vi "_findOpenStorage.vi"(4 "error in (no error)":errorcluster, 6 "Storage type":string="USI", 7 "Storage location":path) -> (0 "error out":errorcluster, 3 "storage refnum":refnum<k20>)   [LabVIEW 2020]
uses:
  <resource>/objmgr/Storage.rc
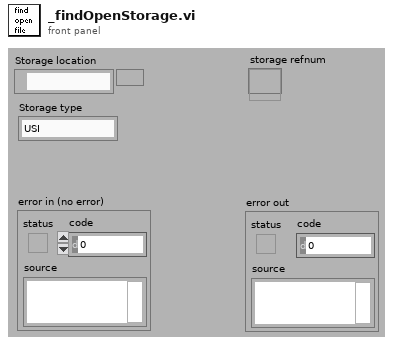
[diagram p1: front panel]
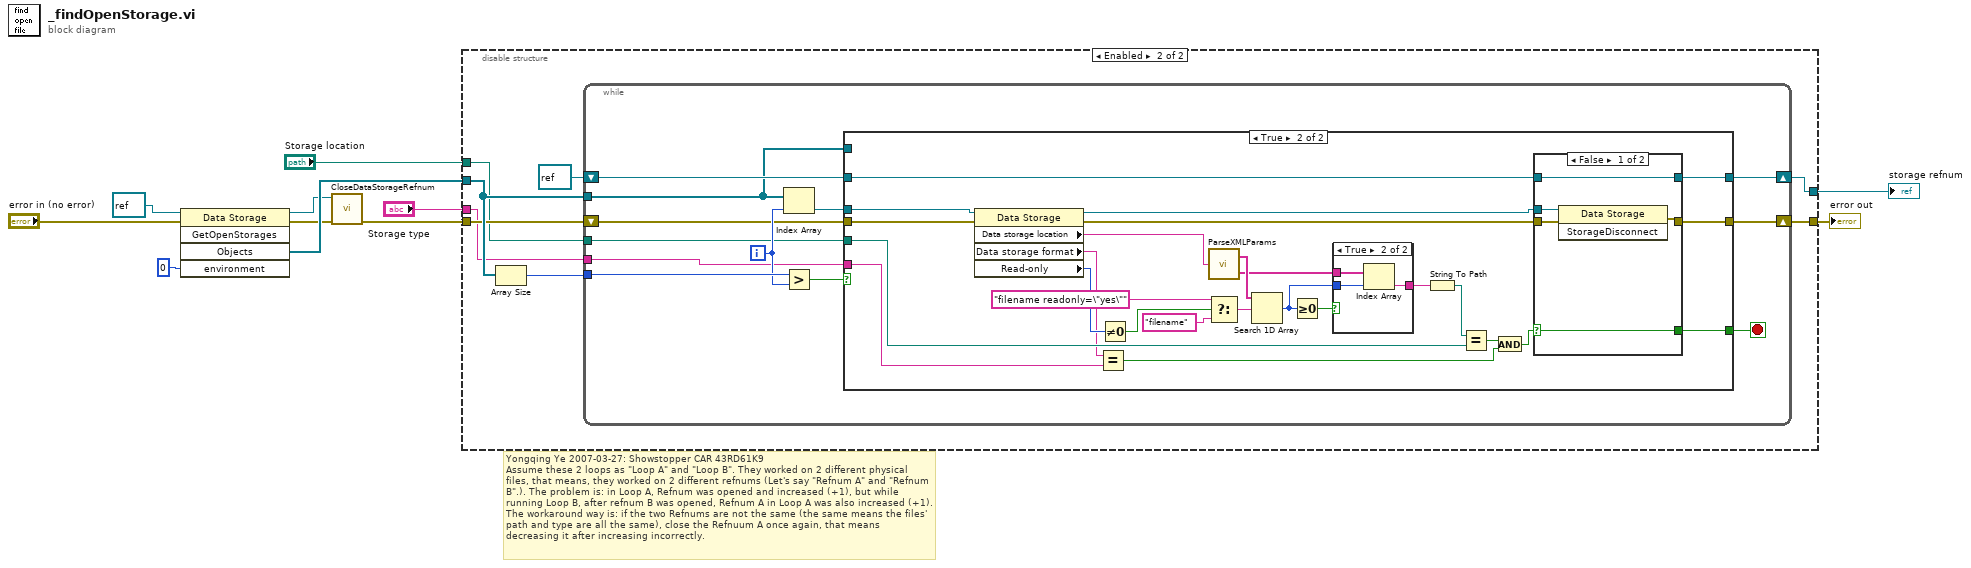
[diagram p0: block diagram]
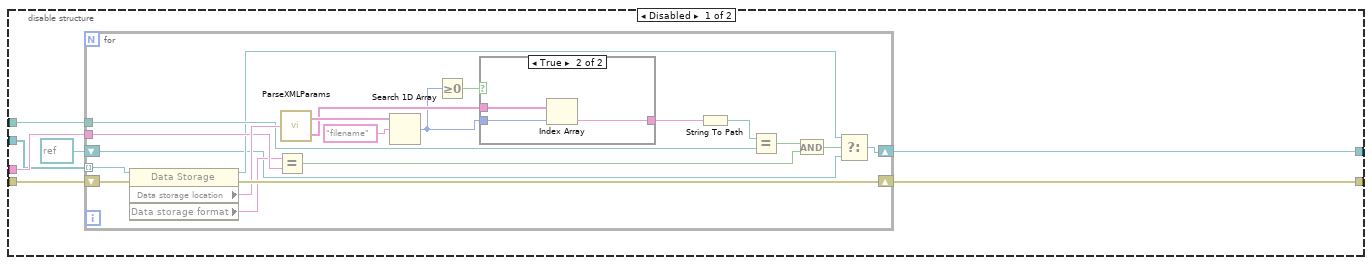
[diagram p2: hidden frame]
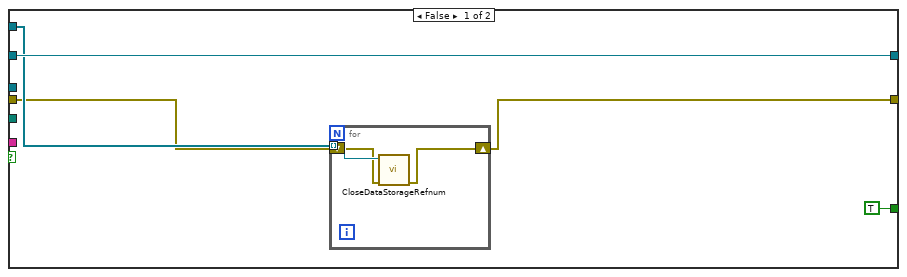
[diagram p4: hidden frame]
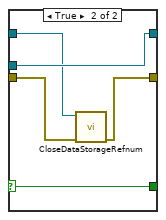
[diagram p6: hidden frame]
diagram:
  # "Yongqing Ye 2007-03-27: Showstopper CAR 43RD61K9\nAssume these 2 loops as \"Loop A\" and \"Loop B\". They worked on 2 different physical files, that means, they worked on 2 different refnums (Let's say \"Refnum A\" and \"Refnum B\".). The problem is: in Loop A, Refnum was opened and increased (+1), but while running Loop B, after refnum B was opened, Refnum A in Loop A was also increased (+1). The workaround way is: if the two Refnums are not the same (the same means the files' path and type are all the same), close the Refnuum A once again, that means decreasing it after increasing incorrectly."
  n1 = invoke class="Data Storage" method="GetOpenStorages"(reference=refnum<k20> refnum, error in="error in (no error)", "environment"=0) -> (reference out=w3:refnum<k20>, error out=w2:errorcluster, "Objects"=w6:refnum<k20>[])  [unwired: 2 in, 2 out]
  n2 = call "CloseDataStorageRefnum.vi"("error in (no error)"=w2, "reference"=w3) -> ("error out"=w1:errorcluster)  [unwired: 9 in]
  n3 = disable-structure shown="Enabled" {
    disable-tunnel: [w18 w42] -> w11
    disable-tunnel: "Storage type" -> [w17 w44]
    disable-tunnel: "Storage location" -> [w16 w45]
    disable-tunnel: [w15 w43] -> w7
    disable-tunnel: w1 -> [w14 w46]
    disable-tunnel: w6 -> [w13 w48]
    frame Disabled {
      n4 = for {
        tunnel: w13 -> [w38] mode=indexing
        shift-right: [w36] -> w18
        shift-left: w14 -> [w37]
        tunnel: w16 -> [w27]
        tunnel: w17 -> [w26]
        shift-right: [w19] -> w15
        shift-left: refnum<k20> refnum ("reference") -> [w20]
        n5 = property class="Data Storage"(reference=w38, error in=w37) -> (reference out=w21:refnum<k20>, error out=w36:errorcluster, "Data storage location"=w30:string, "Data storage format"=w25:string)
        n6 = Equal?(x=w25, y=w26) -> (x = y?=w24:bool)
        n7 = call "ParseXMLParams.vi"("Parameter String"=w30) -> ("Names"=w35:string[], "Values"=w32:string[])
        n8 = Search 1D Array(1D array=w35, element="filename") -> (index of element=w31:i32)  [unwired: 1 in]
        n9 = Greater Or Equal To 0?(x=w31) -> (x >= 0?=w33:bool)
        n10 = case shown="True" w33 {
          tunnel: w32 -> [_ w41]
          tunnel: w31 -> [_ w40]
          tunnel: [_ w39] -> w29
          frame False {
          }
          frame True {
            n11 = Index Array(array=w41, index=w40) -> (element=w39:string)
          }
        }
        n12 = String To Path(string=w29) -> (path=w28:path)
        n13 = Equal?(x=w28, y=w27) -> (x = y?=w23:bool)
        n14 = And(x=w23, y=w24) -> (x .and. y?=w22:bool)
        n15 = Select(t=w21, s=w22, f=w20) -> (s? t:f=w19:refnum<k20>)
      }
    }
    frame Enabled {
      n16 = Array Size(array=w48) -> (size(s)=w49:i32)
      n17 = while {
        tunnel: w49 -> [w61]
        tunnel: w48 -> [w50]
        shift-right: [w51] -> w43
        shift-left: refnum<k20> refnum ("reference") -> [w57]
        tunnel: w45 -> [w55]
        tunnel: w44 -> [w54]
        shift-right: [w52] -> w42
        shift-left: w46 -> [w56]
        i -> [w59]
        stop <- w53 stop-if-true
        n18 = Index Array(array=w50, index=w59) -> (element=w58:refnum<k20>)
        n19 = Greater?(x=w61, y=w59) -> (0:w60:bool)
        n20 = case shown="True" w60 {
          tunnel: w58 -> [_ w76]
          tunnel: w57 -> [w65 w89]
          tunnel: w56 -> [w63 w75]
          tunnel: w55 -> [_ w93]
          tunnel: w54 -> [_ w92]
          tunnel: [TRUE w87] -> w53
          tunnel: [w62 w88] -> w52
          tunnel: [w65 w90] -> w51
          tunnel: w50 -> [w64 _]
          frame False {
            n21 = for {
              tunnel: w64 -> [w69] mode=indexing
              shift-right: [w67] -> w62
              shift-left: w63 -> [w68]
              n22 = call "CloseDataStorageRefnum.vi"("error in (no error)"=w68, "reference"=w69) -> ("error out"=w67:errorcluster)  [unwired: 9 in]
            }
          }
          frame True {
            n23 = property class="Data Storage"(reference=w76, error in=w75) -> (reference out=w74:refnum<k20>, error out=w73:errorcluster, "Data storage location"=w72:string, "Data storage format"=w70:string, "Read-only"=w71:i32)
            n24 = Equal?(x=w70, y=w92) -> (x = y?=w95:bool)
            n25 = Not Equal To 0?(x=w71) -> (x != 0?=w79:bool)
            n26 = call "ParseXMLParams.vi"("Parameter String"=w72) -> ("Names"=w86:string[], "Values"=w84:string[])
            n27 = Select(t="filename readonly=\"yes\"", s=w79, f="filename" ("element")) -> (s? t:f=w80:string)
            n28 = Search 1D Array(1D array=w86, element=w80) -> (index of element=w83:i32)  [unwired: 1 out]
            n29 = Greater Or Equal To 0?(x=w83) -> (x >= 0?=w85:bool)
            n30 = case shown="True" w85 {
              tunnel: w84 -> [_ w98]
              tunnel: w83 -> [_ w97]
              tunnel: [_ w96] -> w78
              frame False {
              }
              frame True {
                n31 = Index Array(array=w98, index=w97) -> (element=w96:string)
              }
            }
            n32 = String To Path(string=w78) -> (path=w77:path)
            n33 = Equal?(x=w77, y=w93) -> (x = y?=w94:bool)
            n34 = And(x=w94, y=w95) -> (x .and. y?=w91:bool)
            n35 = case shown="False" w91 {
              selector: w91 -> [w102 w107]
              tunnel: w74 -> [w101 w108]
              tunnel: [w103 w108] -> w90
              tunnel: w73 -> [w100 w105]
              tunnel: w89 -> [w103 w106]
              tunnel: [w99 w104] -> w88
              tunnel: [w102 w107] -> w87
              frame False {
                n36 = invoke class="Data Storage" method="StorageDisconnect"(reference=w101, error in=w100) -> (error out=w99:errorcluster)  [unwired: 1 in, 2 out]
              }
              frame True {
                n37 = call "CloseDataStorageRefnum.vi"("error in (no error)"=w105, "reference"=w106) -> ("error out"=w104:errorcluster)  [unwired: 9 in]
              }
            }
          }
        }
      }
    }
  }
  "error out" <- w11
  "storage refnum" <- w7
